vi "Solve1.vi"(8 "Error In":errorcluster, 11 "object in":refnum<class "2021_4.lvclass">) -> (0 "Error Out":errorcluster, 2 "Result":u64, 3 "object out":refnum<class "2021_4.lvclass">)   [LabVIEW 2020, in "2021_4.lvclass"]
uses:
  2021_4.lvclass
  2021_4.lvclass/2021_4.ctl
panel:
  out "Board":i32
  out "Boards":bool[][][](array[boolean])
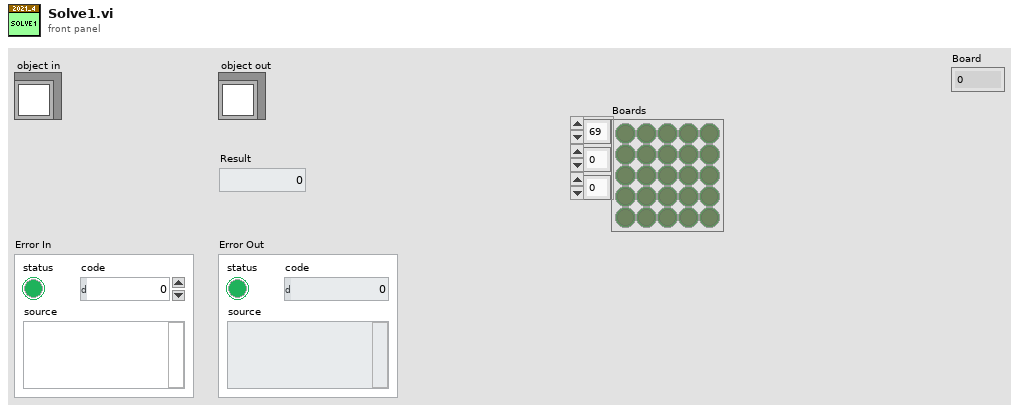
[diagram p1: front panel]
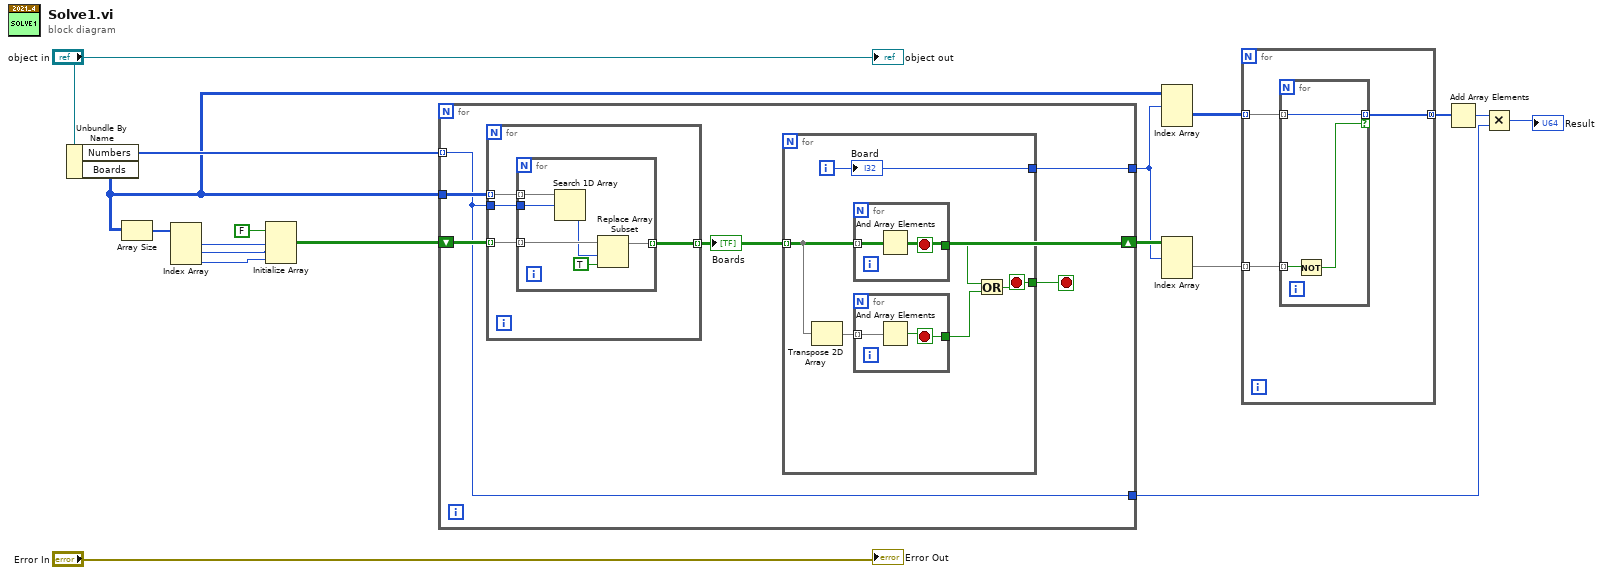
[diagram p0: block diagram]
diagram:
  n1 = Unbundle By Name("object in") -> ("Numbers"=w11:u32[], "Boards"=w9:i32[][][])
  n2 = Array Size(array=w9) -> (size(s)=w16:i32[])
  n3 = Index Array(array=w16) -> (element #1=w15:i32, element #2=w14:i32, element #3=w13:i32)  [unwired: 3 in]
  n4 = Initialize Array(FALSE, w15, w14, w13) -> (w10:bool[][][])
  n5 = for {
    tunnel: w11 -> [w19] mode=indexing
    tunnel: w9 -> [w23]
    shift-right: [w22] -> w7
    shift-left: w10 -> [w24]
    tunnel: [w21] -> w6
    tunnel: [w19] -> w2
    stop <- w20 stop-if-true
    n6 = for {
      tunnel: w24 -> [w37] mode=indexing
      tunnel: w23 -> [w38] mode=indexing
      tunnel: w19 -> [w36]
      tunnel: [w35] -> w22 mode=indexing
      n7 = for {
        tunnel: w38 -> [w44] mode=indexing
        tunnel: w37 -> [w42] mode=indexing
        tunnel: w36 -> [w43]
        tunnel: [w39] -> w35 mode=indexing
        n8 = Search 1D Array(1D array=w44, element=w43) -> (index of element=w41:i32)  [unwired: 1 in]
        n9 = Replace Array Subset(array=w42, new element=TRUE ("new element/subarray"), index=w41) -> (w39:bool[])
      }
    }
    "Boards" <- w22
    n10 = for {
      tunnel: w22 -> [w30] mode=indexing
      tunnel: [w26] -> w21
      tunnel: [w25] -> w20
      i -> [w26]
      stop <- w25 stop-if-true
      n11 = Transpose 2D Array(2D array=w30) -> (transposed array=w29:bool[][])
      n12 = for {
        tunnel: w30 -> [w34] mode=indexing
        tunnel: [w33] -> w28
        stop <- w33 stop-if-true
        n13 = And Array Elements(Boolean array=w34) -> (logical AND=w33:bool)
      }
      n14 = for {
        tunnel: w29 -> [w32] mode=indexing
        tunnel: [w31] -> w27
        stop <- w31 stop-if-true
        n15 = And Array Elements(Boolean array=w32) -> (logical AND=w31:bool)
      }
      n16 = Or(x=w28, y=w27) -> (x .or. y?=w25:bool)
      "Board" <- w26
    }
  }
  n17 = Index Array(array=w9, index (dim 0)=w6) -> (element=w8:i32[][])  [unwired: 2 in]
  n18 = Index Array(array=w7, index (dim 0)=w6) -> (element=w5:bool[][])  [unwired: 2 in]
  n19 = for {
    tunnel: w8 -> [w47] mode=indexing
    tunnel: w5 -> [w46] mode=indexing
    tunnel: [w45] -> w4 mode=concatenating
    n20 = for {
      tunnel: w47 -> [w50] mode=indexing
      tunnel: w46 -> [w49] mode=indexing
      tunnel: [w50] -> w45 mode=indexing if=w48
      n21 = Not(x=w49) -> (.not. x?=w48:bool)
    }
  }
  n22 = Add Array Elements(numeric array=w4) -> (sum=w3:i32)
  n23 = Multiply(x=w3, y=w2) -> (x*y=→"Result":u32)
  "Error Out" <- "Error In"
  "object out" <- "object in"
